vi "Plot resize horizontal.vi"(8 "error in (no error)":errorcluster, 11 "Refs":T1) -> (0 "error out":errorcluster)   [LabVIEW 2021, in "RocketPlot.lvlib"]
uses:
  RocketPlot.lvlib
  TypeDefs/Plot UI references.ctl
  Classes/RocketPlotHandle/RocketPlotHandle.lvclass
  <userlib>/bjustice/TipStripOOPanel/Classes/TipPanelHandle/TipPanelHandle.lvclass
  TypeDefs/Plot top row.ctl
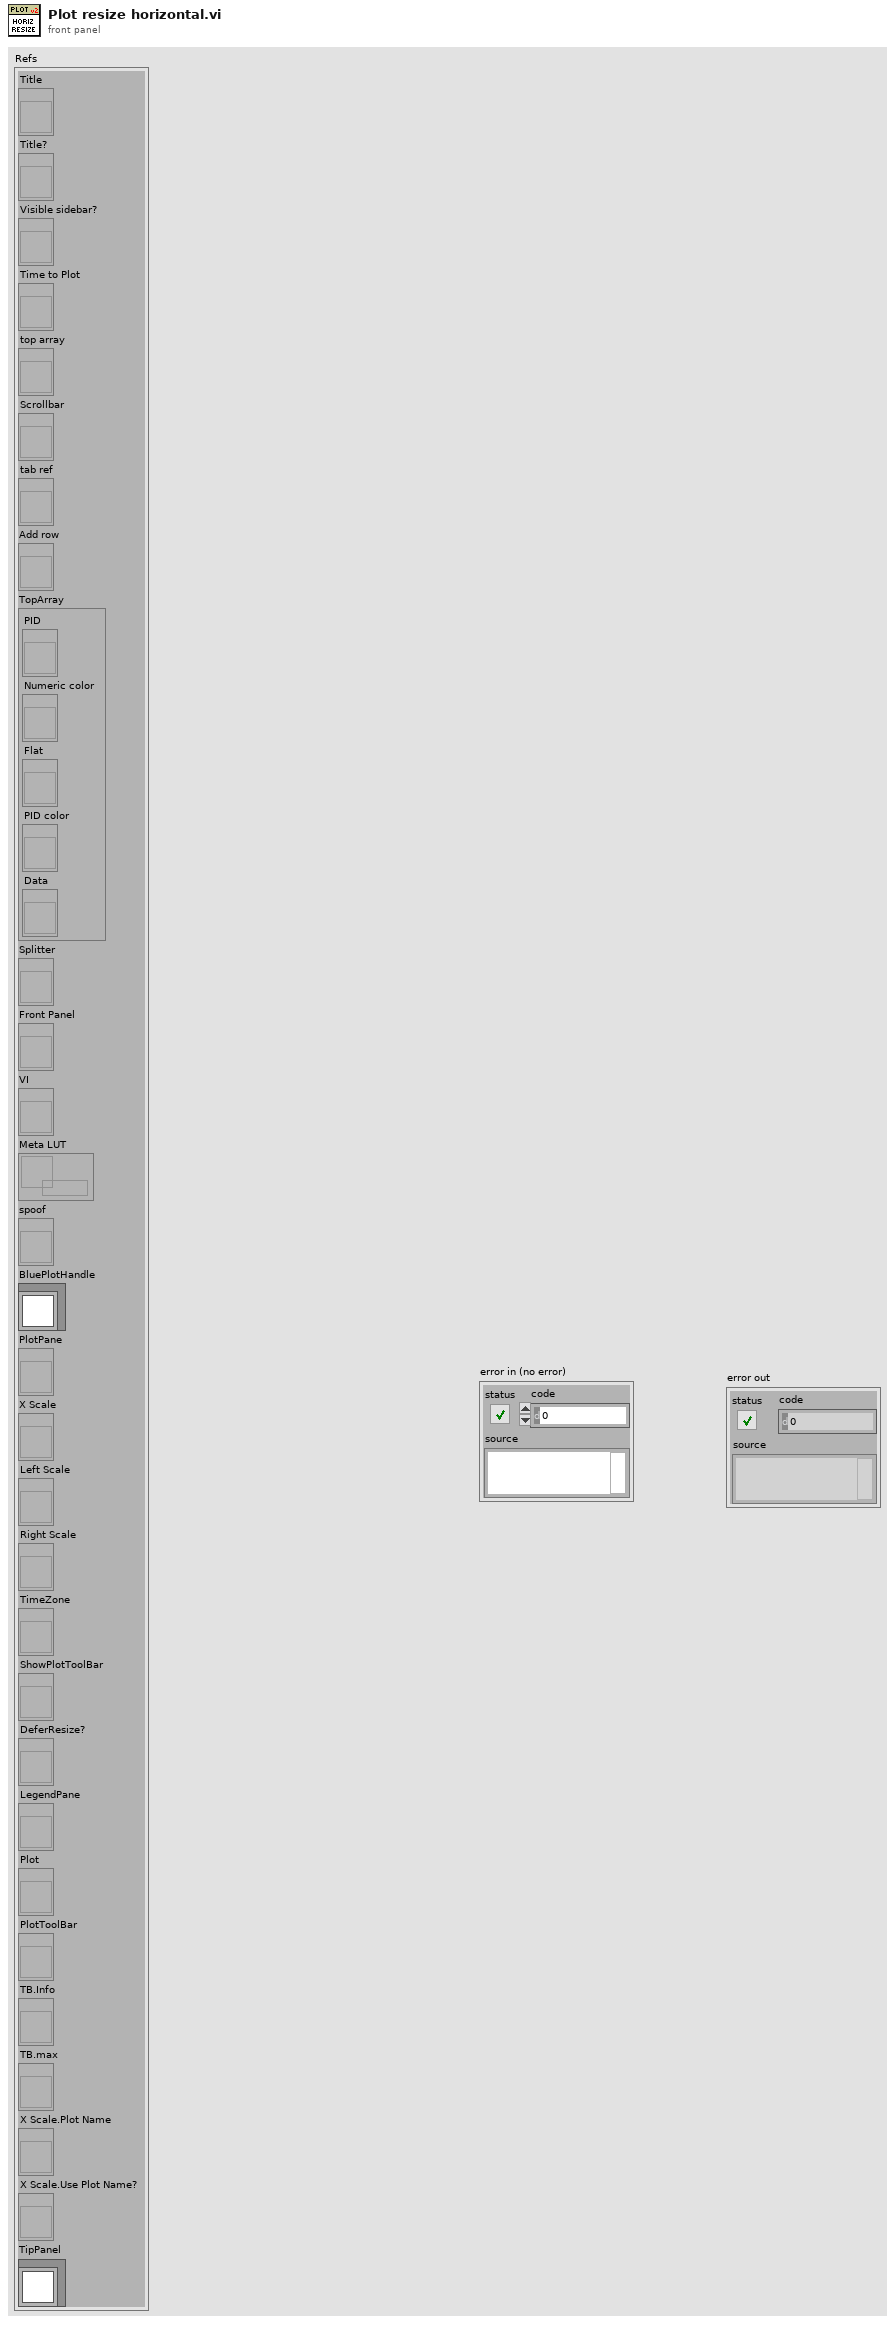
[diagram p1: front panel]
types:
  T1 = typedef "RocketPlot.lvlib/Plot UI references.ctl" = cluster{"Title":refnum<vi>, "Title?":refnum<vi>, "Visible sidebar?":refnum<vi>, "Time to Plot":refnum<vi>, "top array":refnum<vi>, "Scrollbar":refnum<vi>, "tab ref":refnum<vi>, "Add row":refnum<vi>, "TopArray":cluster{"PID":refnum<vi>, "Numeric color":refnum<vi>, "Flat":refnum<vi>, "PID color":refnum<vi>, "Data":refnum<vi>}, "Splitter":refnum<vi>, "Front Panel":refnum<vi>, "VI":refnum<vi>, "Meta LUT":refnum<data-value>, "spoof":refnum<vi>, "BluePlotHandle":refnum<class "RocketPlotHandle.lvclass">, "PlotPane":refnum<vi>, "X Scale":refnum<vi>, "Left Scale":refnum<vi>, "Right Scale":refnum<vi>, "TimeZone":refnum<vi>, "ShowPlotToolBar":refnum<vi>, "DeferResize?":refnum<vi>, "LegendPane":refnum<vi>, "Plot":refnum<vi>, "PlotToolBar":refnum<vi>, "TB.Info":refnum<vi>, "TB.max":refnum<vi>, "X Scale.Plot Name":refnum<vi>, "X Scale.Use Plot Name?":refnum<vi>, "TipPanel":refnum<class "TipPanelHandle.lvclass">}
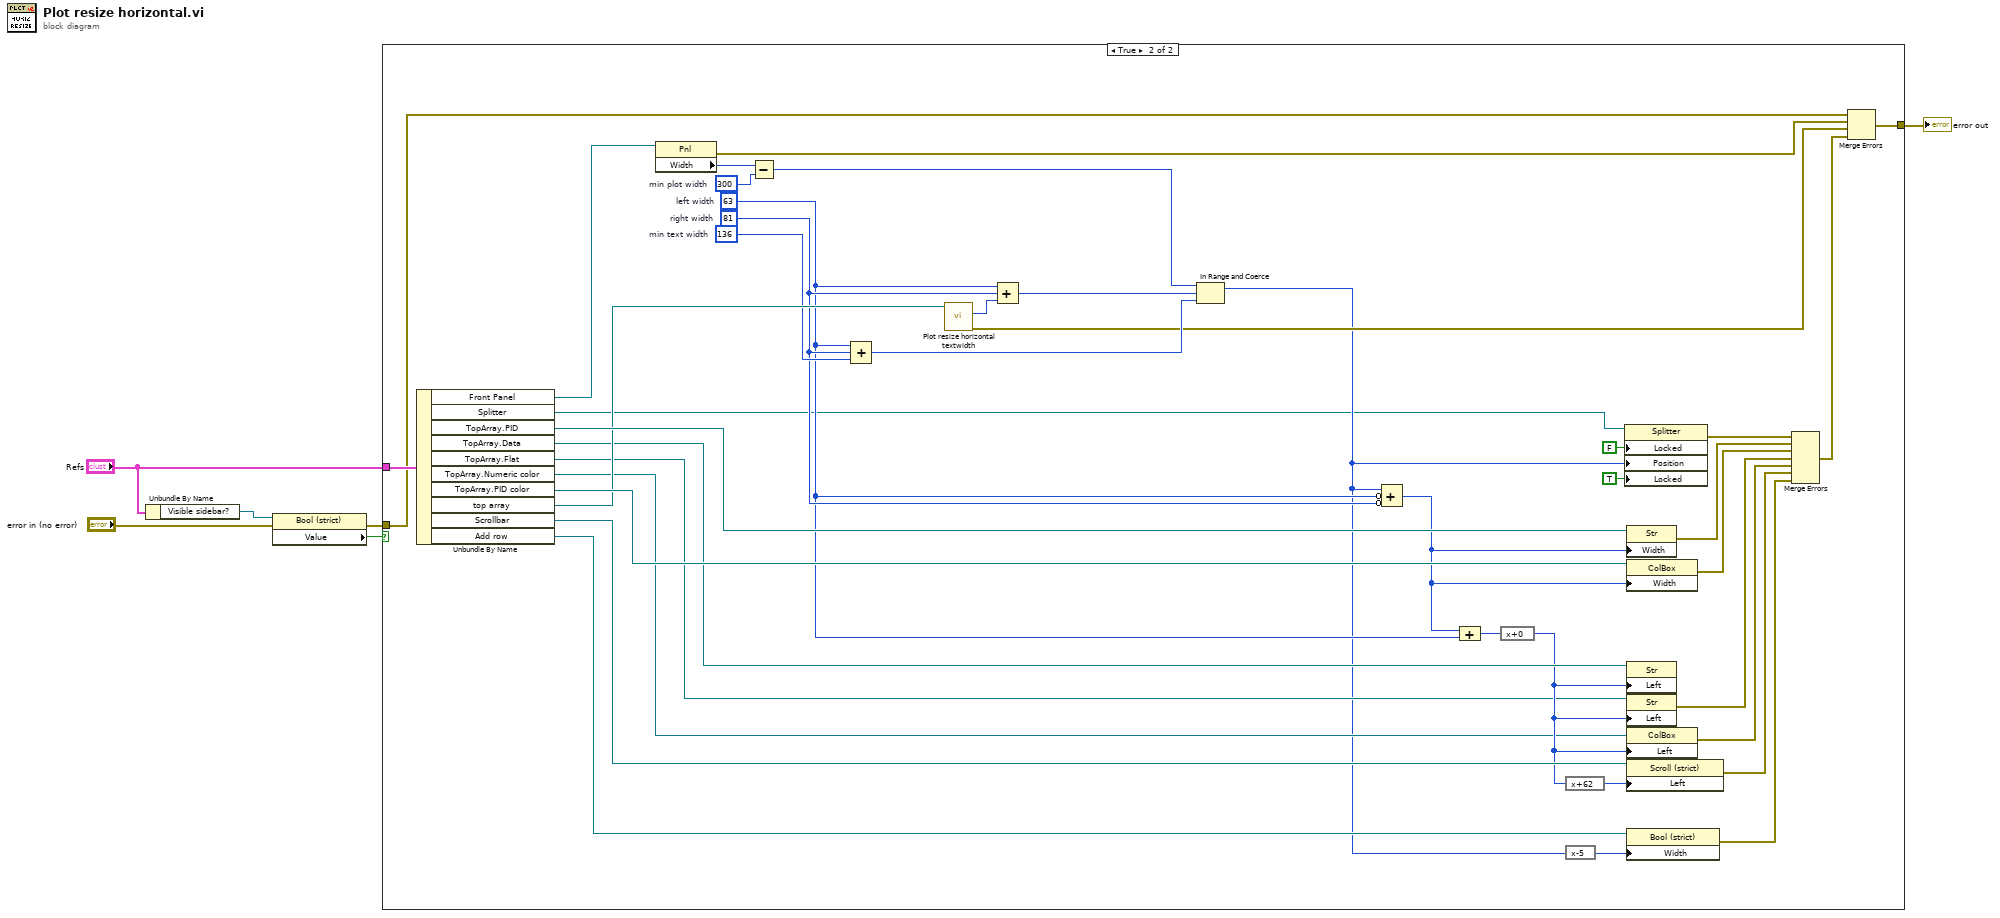
[diagram p0: block diagram]
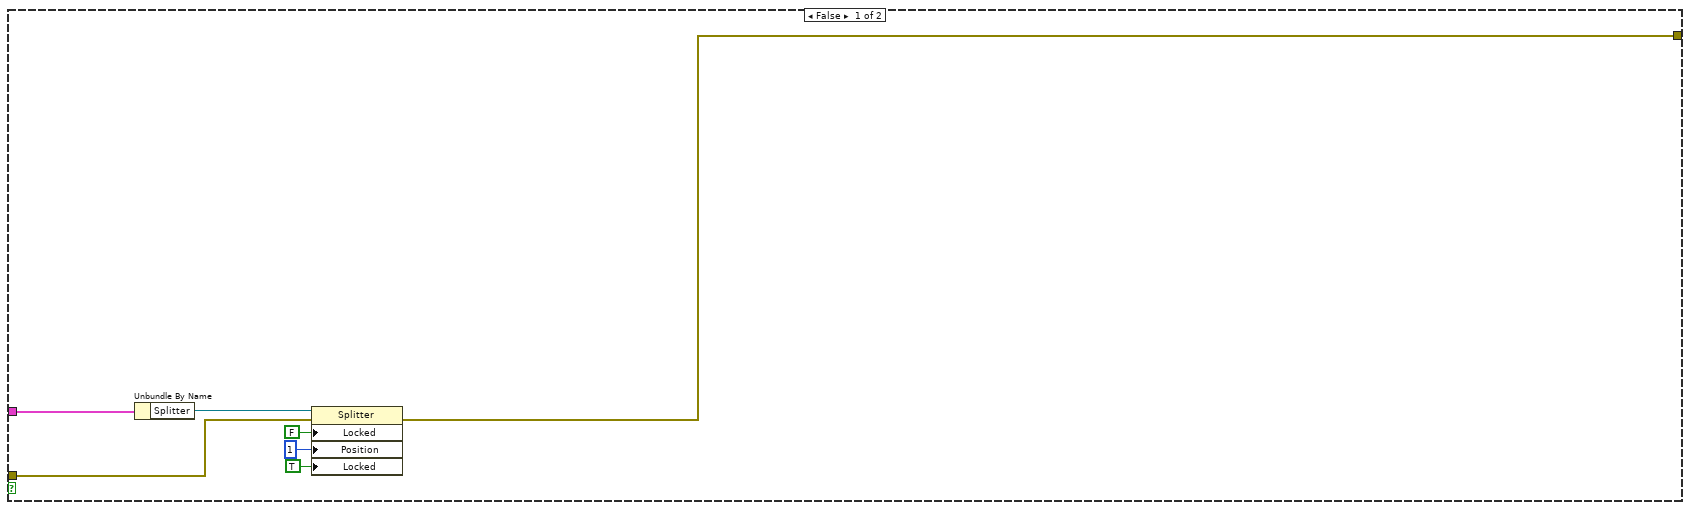
[diagram p2: hidden frame]
diagram:
  n1 = Unbundle By Name("Refs") -> ("Visible sidebar?"=w6:refnum<vi>)
  n2 = property class="Bool (strict)"(reference=w6, error in="error in (no error)") -> (error out=w3:errorcluster, "Value"=w4:bool)  [unwired: 1 out]
  n3 = case shown="True" w4 {
    tunnel: "Refs" -> [w13 w53]
    tunnel: [w11 w26] -> w1
    tunnel: w3 -> [w10 w15]
    frame False {
      n4 = Unbundle By Name(w13) -> ("Splitter"=w12:refnum<vi>)
      n5 = property class="Splitter"(reference=w12, error in=w10, "Locked"=FALSE ("Splitter Position Locked"), "Position"=1 ("Splitter Position"), "Locked"=TRUE ("Splitter Position Locked")) -> (error out=w11:errorcluster)  [unwired: 1 out]
    }
    frame True {
      w48 = u32 136  # min text width
      w38 = u32 300  # min plot width
      w47 = u32 81  # right width
      w46 = u32 63  # left width
      n6 = Unbundle By Name(w53) -> ("Front Panel"=w39:refnum<vi>, "Splitter"=w14:refnum<vi>, "TopArray.PID"=w50:refnum<vi>, "TopArray.Data"=w24:refnum<vi>, "TopArray.Flat"=w22:refnum<vi>, "TopArray.Numeric color"=w21:refnum<vi>, "TopArray.PID color"=w52:refnum<vi>, "top array"=w49:refnum<vi>, "Scrollbar"=w51:refnum<vi>, "Add row"=w25:refnum<vi>)
      n7 = property class="Pnl"(reference=w39) -> (error out=w36:errorcluster, "Width"=w40:u32)  [unwired: 1 in, 1 out]
      n8 = Subtract(x=w40, y=w38) -> (x-y=w37:u32)
      n9 = Compound Arithmetic op=unknown(w46, w47, w48) -> (w41:u32)
      n10 = call "Plot resize horizontal textwidth.vi"("top array"=w49) -> ("error out"=w35:errorcluster, "full textbox width"=w17:i16)  [unwired: 9 in]
      n11 = Compound Arithmetic op=unknown(w46, w47, w17) -> (w16:u32)
      n12 = In Range and Coerce(upper limit=w37, x=w16, lower limit=w41) -> (coerced(x)=w20:u32)  [unwired: 1 out]
      n13 = Compound Arithmetic op=ADD(w20, invert w46, invert w47) -> (w43:u32)
      n14 = Compound Arithmetic op=ADD(w43, w46) -> (w42:u32)
      n15 = expression code="x+0"(w42) -> (w23:u32)
      n16 = expression code="x+62"(w23) -> (w45:u32)
      n17 = expression code="x-5"(w20) -> (w44:u32)
      n18 = property class="Splitter"(reference=w14, "Locked"=FALSE ("Splitter Position Locked"), "Position"=w20, "Locked"=TRUE ("Splitter Position Locked")) -> (error out=w34:errorcluster)  [unwired: 1 in, 1 out]
      n19 = property class="Str"(reference=w50, "Width"=w43) -> (error out=w33:errorcluster)  [unwired: 1 in, 1 out]
      n20 = property class="ColBox"(reference=w52, "Width"=w43) -> (error out=w32:errorcluster)  [unwired: 1 in, 1 out]
      n21 = property class="Str"(reference=w24, "Left"=w23) -> ()  [unwired: 1 in, 2 out]
      n22 = property class="Str"(reference=w22, "Left"=w23) -> (error out=w31:errorcluster)  [unwired: 1 in, 1 out]
      n23 = property class="ColBox"(reference=w21, "Left"=w23) -> (error out=w30:errorcluster)  [unwired: 1 in, 1 out]
      n24 = property class="Scroll (strict)"(reference=w51, "Left"=w45) -> (error out=w29:errorcluster)  [unwired: 1 in, 1 out]
      n25 = property class="Bool (strict)"(reference=w25, "Width"=w44) -> (error out=w28:errorcluster)  [unwired: 1 in, 1 out]
      n26 = Merge Errors(w34, w33, w32, w31, w30, w29, w28) -> (w27:errorcluster)
      n27 = Merge Errors(w15, w36, w35, w27) -> (w26:errorcluster)
    }
  }
  "error out" <- w1
